vi "CLSUIP_GetNamedUnbundler.vi"(8 "error in (no error)":errorcluster, 11 "VI Refnum":refnum<vi>) -> (0 "error out":errorcluster, 2 "NmdBundler Ref":refnum<vi>, 3 "VI Refnum out":refnum<vi>)   [LabVIEW 2021, in "MemberVICreation.lvlib"]
uses:
  <resource>/Framework/Providers/LVClassLibrary/NewAccessors/MemberVICreation.lvlib
  <vilib>/Utility/traverseref.llb/TRef TravTarget.ctl
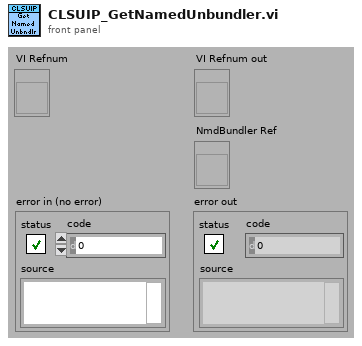
[diagram p1: front panel]
types:
  T1 = typedef "TRef TravTarget.ctl" = enum16{"FP", "BD", "Other"}
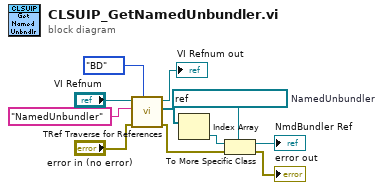
[diagram p0: block diagram]
diagram:
  w11 = refnum<vi> refnum  # NamedUnbundler
  n1 = call <vilib>:"TRef Traverse for References.vi"("Traverse Target"=TRef_TravTarget."BD", "error in (no error)"="error in (no error)", "Class Name"="NamedUnbundler" ("y"), "VI Refnum"="VI Refnum") -> ("error out"=w3:errorcluster, "References"=w4:refnum<vi>[], "dup VI Refnum"=→"VI Refnum out":refnum<vi>)  [unwired: 1 in, 4 out]
  n2 = Index Array(array=w4) -> (element=w2:refnum<vi>)  [unwired: 1 in]
  n3 = To More Specific Class(target class=w11, reference=w2, error in=w3) -> (specific class reference=→"NmdBundler Ref":refnum<vi>, error out=→"error out":errorcluster)
